vi "csm_lumikki_instron_moveToSetpoint_5.vi"(7 "channelInt":i32=1, 8 "rampRate":dbl=1.0, 9 "rampAmplitude":dbl=1.0, 10 "setPointTime":dbl=1.0, 11 "setPoint":dbl=1.0) -> (0 "rampRateOut":dbl, 1 "rampAmplitudeOut":dbl, 2 "setpointTimeOut":dbl, 3 "setpointOut":dbl, 4 "iAmBusyCommandNotExecuted":bool, 5 "channelIntOut":i32)   [LabVIEW 2009]
panel:
  in  "channelInt 2":i32=1
  in  "rampRate 2":dbl=1.0
  in  "rampAmplitude 2":dbl=1.0
  in  "setPointTime 2":dbl=1.0
  in  "setPoint 2":dbl=1.0
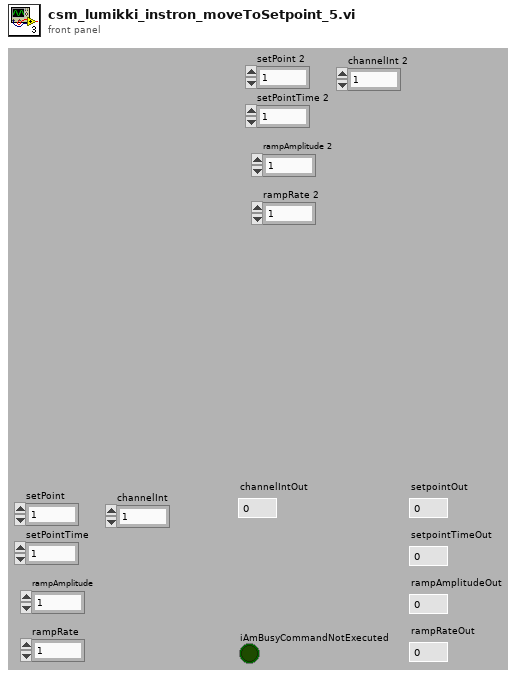
[diagram p1: front panel]
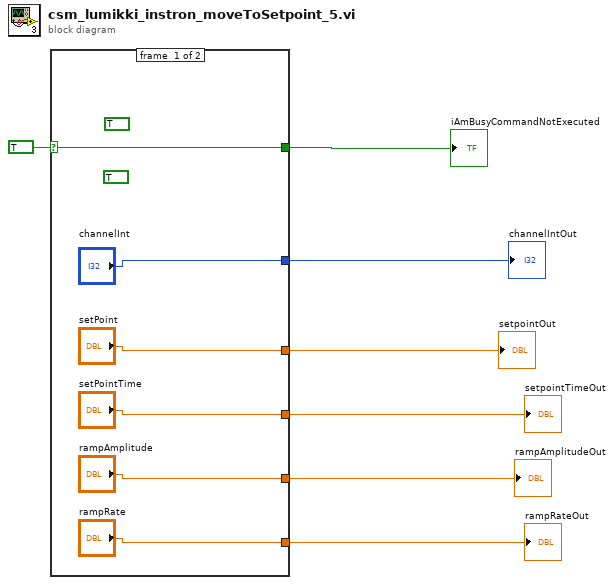
[diagram p0: block diagram]
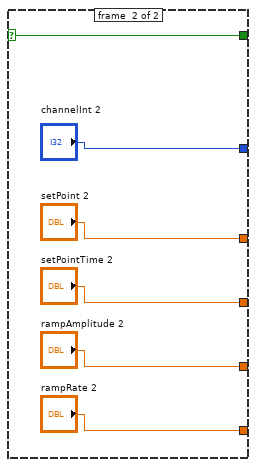
[diagram p2: hidden frame]
diagram:
  n1 = case shown="True" TRUE {
    selector: TRUE -> [w13 w19]
    tunnel: [w13 w19] -> w7
    tunnel: ["channelInt" "channelInt 2"] -> w6
    tunnel: ["setPoint" "setPoint 2"] -> w5
    tunnel: ["setPointTime" "setPointTime 2"] -> w1
    tunnel: ["rampAmplitude" "rampAmplitude 2"] -> w4
    tunnel: ["rampRate" "rampRate 2"] -> w3
    frame #0 {
      (unwired) TRUE ("Busy")
      (unwired) TRUE ("Busy")
    }
    frame #1 {
    }
  }
  "iAmBusyCommandNotExecuted" <- w7
  "channelIntOut" <- w6
  "setpointOut" <- w5
  "setpointTimeOut" <- w1
  "rampAmplitudeOut" <- w4
  "rampRateOut" <- w3
